vi "UTIL Progress Bar Close.vi"(8 "error in (no error)":errorcluster, 11 "reference in":refnum<vi>) -> (0 "error out":errorcluster)   [LabVIEW 2019]
doc: "10/01/2010\n\nNational Analytics (TLE)\n\nClose the progress bar."
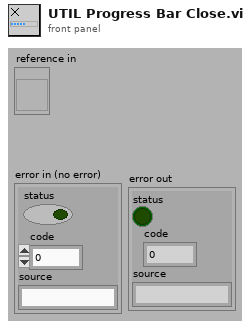
[diagram p1: front panel]
types:
  T1 = enum32{"Invalid", "Standard", "Closed", "Hidden", "Minimized", "Maximized"}
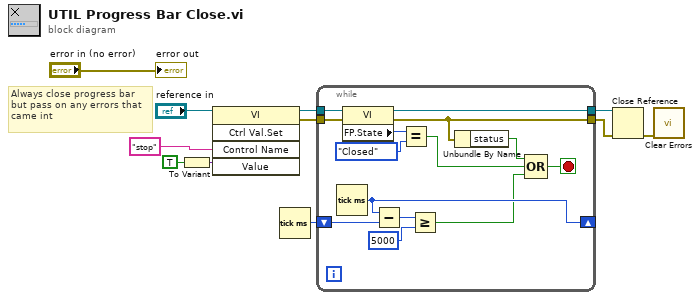
[diagram p0: block diagram]
diagram:
  # "Always close progress bar\nbut pass on any errors that\ncame int"
  n1 = To Variant(anything=TRUE) -> (Variant=w8:variant)
  n2 = invoke class="VI" method="Ctrl Val.Set"(reference="reference in", "Control Name"="stop", "Value"=w8) -> (reference out=w6:refnum<vi>, error out=w4:errorcluster)  [unwired: 2 in, 3 out]
  n3 = Tick Count (ms)() -> (millisecond timer value=w1:u32)
  n4 = while {
    tunnel: w6 -> [w25]
    tunnel: [w24] -> w5
    tunnel: w4 -> [w21]
    tunnel: [w20] -> w3
    shift-right: [w15] -> _
    shift-left: w1 -> [w16]
    stop <- w18 stop-if-true
    n5 = Tick Count (ms)() -> (millisecond timer value=w15:u32)
    n6 = property class="VI"(reference=w25, error in=w21) -> (reference out=w24:refnum<vi>, error out=w20:errorcluster, "FP.State"=w23:T1)
    n7 = Subtract(x=w15, y=w16) -> (x-y=w14:u32)
    n8 = Equal?(x=w23, y=T1."Closed") -> (x = y?=w19:bool)
    n9 = Greater Or Equal?(x=w14, y=u32 5000) -> (x >= y?=w12:bool)
    n10 = Unbundle By Name(w20) -> ("status"=w17:bool)
    n11 = Compound Arithmetic op=OR(w17, w19, w12) -> (w18:bool)
  }
  n12 = Close Reference(reference=w5, error in (no error)=w3) -> (error out=w2:errorcluster)
  n13 = call <vilib>:"Clear Errors.vi"("error in (no error)"=w2) -> ()  [unwired: 5 in, 2 out]
  "error out" <- "error in (no error)"
